vi "RP Transmit Data.vi"   [LabVIEW 2019]
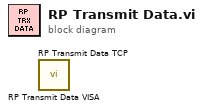
[diagram p0: block diagram]
diagram:
  n1 = call "RP Transmit Data VISA.vi"() -> ()  [unwired: 10 in, 2 out]
  n2 = call "RP Transmit Data TCP.vi"() -> ()  [unwired: 10 in, 2 out]
